vi "Example5-Encapsulation.vi"() -> ()   [LabVIEW 2021]
doc: "Example of object encapsulation in LabVIEW. Comments in Polish."
uses:
  Droid/Droid.lvclass
  Astromech droid/Astromech droid.lvclass
  BB-Series/BB-Series.lvclass
  MedicalDroid/MedicalDroid.lvclass
  BactaTank/BactaTank.lvclass
  BattleDroid/BattleDroid.lvclass
  B1/B1.lvclass
panel:
  out "Output DROID data":cluster{"ID":string, "Active":bool}
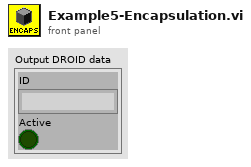
[diagram p1: front panel]
types:
  T1 = cluster{"Mode ":enum16{"GUARD", "RECON", "ATTACK ", "MAINTAINCE"}, "Enviroment Info":variant, "Mission Goals":string[], "DataAboutEnemy":map{string, i32}}
  T2 = enum16{"GUARD", "RECON", "ATTACK ", "MAINTAINCE"}
  T3 = enum16{"Q-Series", "BB-Series", "C-Series", "R-Series"}
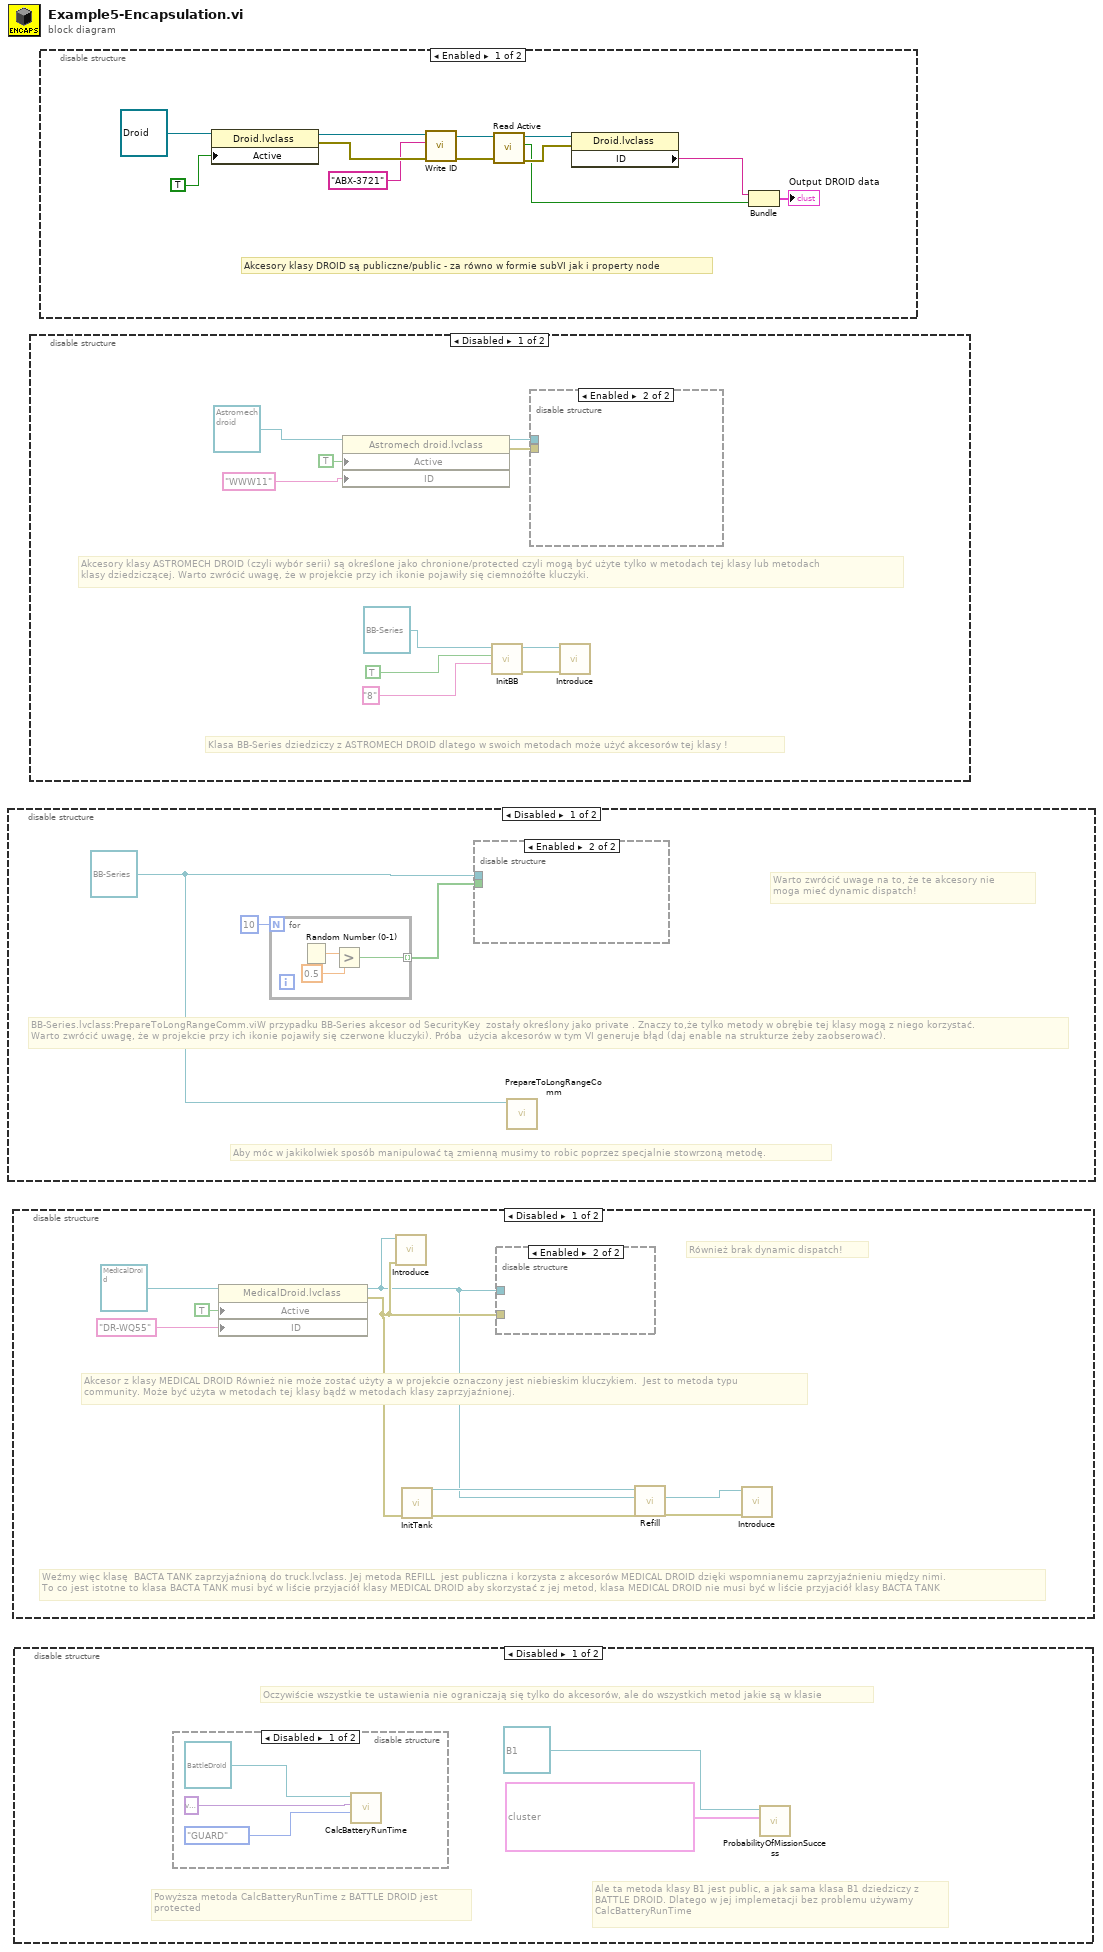
[diagram p0: block diagram]
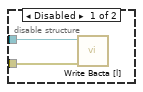
[diagram p4: hidden frame]
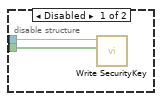
[diagram p6: hidden frame]
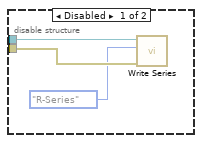
[diagram p8: hidden frame]
diagram:
  n1 = disable-structure shown="Disabled" {
    frame Disabled {
      w1 = refnum<class "BB-Series.lvclass"> refnum ("BB-Series in")
      # "Warto zwrócić uwage na to, że te akcesory nie \nmoga mieć dynamic dispatch!"
      # "Aby móc w jakikolwiek sposób manipulować tą zmienną musimy to robic poprzez specjalnie stowrzoną metodę."
      # "BB-Series.lvclass:PrepareToLongRangeComm.viW przypadku BB-Series akcesor od SecurityKey  zostały określony jako private . Znaczy to,że tylko metody w obrębie tej klasy mogą z niego korzystać. \nWarto zwrócić uwagę, że w projekcie przy ich ikonie pojawiły się czerwone kluczyki). Próba  użycia akcesorów w tym VI generuje błąd (daj enable na strukturze żeby zaobserować)."
      n2 = for {
        N: 10 -> [_]
        tunnel: [w6] -> w2 mode=indexing
        n3 = Random Number (0-1)() -> (number: 0 to 1=w8:dbl)
        n4 = Greater?(x=w8, y=0.5) -> (0:w6:bool)
      }
      n5 = disable-structure shown="Enabled" {
        disable-tunnel: w1 -> [w5 _]
        disable-tunnel: w2 -> [w4 _]
        frame Disabled {
          n6 = call "Write SecurityKey.vi"("SecurityKey"=w4, "BB-Series in"=w5) -> ()  [unwired: 8 in, 2 out]
        }
        frame Enabled {
        }
      }
      n7 = call "PrepareToLongRangeComm.vi"("BB-Series in"=w1) -> ()  [unwired: 9 in, 2 out]
    }
    frame Enabled {
    }
  }
  n8 = disable-structure shown="Disabled" {
    frame Disabled {
      # "Weźmy więc klasę  BACTA TANK zaprzyjaźnioną do truck.lvclass. Jej metoda REFILL  jest publiczna i korzysta z akcesorów MEDICAL DROID dzięki wspomnianemu zaprzyjaźnieniu między nimi. \nTo co jest istotne to klasa BACTA TANK musi być w liście przyjaciół klasy MEDICAL DROID aby skorzystać z jej metod, klasa MEDICAL DROID nie musi być w liście przyjaciół klasy BACTA TANK"
      # "Również brak dynamic dispatch!"
      # "Akcesor z klasy MEDICAL DROID Również nie może zostać użyty a w projekcie oznaczony jest niebieskim kluczykiem.  Jest to metoda typu\ncommunity. Może być użyta w metodach tej klasy bądź w metodach klasy zaprzyjaźnionej."
      n9 = property class="MedicalDroid.lvclass"(reference=refnum<class "MedicalDroid.lvclass"> refnum ("MedicalDroid.lvclass"), "Active"=TRUE, "ID"="DR-WQ55") -> (reference out=w9:refnum<class "MedicalDroid.lvclass">, error out=w10:errorcluster)  [unwired: 1 in]
      n10 = call-dynamic "Introduce.vi"("Error In"=w10, "MedicalDroid in"=w9) -> ()  [unwired: 8 in, 2 out]
      n11 = call "InitTank.vi"("Error In"=w10) -> ("Error Out"=w15:errorcluster, "BactaTank out"=w14:refnum<class "BactaTank.lvclass">)  [unwired: 9 in]
      n12 = disable-structure shown="Enabled" {
        disable-tunnel: w9 -> [w19 _]
        disable-tunnel: w10 -> [w18 _]
        frame Disabled {
          n13 = call "Write Bacta [l].vi"("error in (no error)"=w18, "MedicalDroid in"=w19) -> ()  [unwired: 8 in, 2 out]
        }
        frame Enabled {
        }
      }
      n14 = call "Refill.vi"("Error In"=w15, "MedicalDroid In"=w9, "BactaTank in"=w14) -> ("Error Out"=w17:errorcluster, "MedicalDroid Out"=w16:refnum<class "MedicalDroid.lvclass">)  [unwired: 6 in, 1 out]
      n15 = call-dynamic "Introduce.vi"("Error In"=w17, "MedicalDroid in"=w16) -> ()  [unwired: 8 in, 2 out]
    }
    frame Enabled {
    }
  }
  n16 = disable-structure shown="Disabled" {
    frame Disabled {
      # "Ale ta metoda klasy B1 jest public, a jak sama klasa B1 dziedziczy z\nBATTLE DROID. Dlatego w jej implemetacji bez problemu używamy\nCalcBatteryRunTime"
      # "Powyższa metoda CalcBatteryRunTime z BATTLE DROID jest \nprotected"
      # "Oczywiście wszystkie te ustawienia nie ograniczają się tylko do akcesorów, ale do wszystkich metod jakie są w klasie"
      n17 = disable-structure shown="Disabled" {
        frame Disabled {
          n18 = call "CalcBatteryRunTime.vi"("Mode"=T2."GUARD", "Enviroment Info"=variant, "BattleDroid In"=refnum<class "BattleDroid.lvclass"> refnum) -> ()  [unwired: 6 in, 3 out]
        }
        frame Enabled {
        }
      }
      n19 = call "ProbabilityOfMissionSuccess.vi"("MissionData"=T1 {"Mode "=enum."GUARD", "Enviroment Info"=variant, "Mission Goals"=[], "DataAboutEnemy"={}}, "B1 In"=refnum<class "B1.lvclass"> refnum) -> ()  [unwired: 7 in, 3 out]
    }
    frame Enabled {
    }
  }
  n20 = disable-structure shown="Disabled" {
    frame Disabled {
      # "Klasa BB-Series dziedziczy z ASTROMECH DROID dlatego w swoich metodach może użyć akcesorów tej klasy !"
      # "Akcesory klasy ASTROMECH DROID (czyli wybór serii) są określone jako chronione/protected czyli mogą być użyte tylko w metodach tej klasy lub metodach\nklasy dziedziczącej. Warto zwrócić uwagę, że w projekcie przy ich ikonie pojawiły się ciemnożółte kluczyki."
      n21 = property class="Astromech droid.lvclass"(reference=refnum<class "Astromech droid.lvclass"> refnum ("Astromech droid.lvclass"), "Active"=TRUE, "ID"="WWW11") -> (reference out=w31:refnum<class "Astromech droid.lvclass">, error out=w30:errorcluster)  [unwired: 1 in]
      n22 = call "InitBB.vi"("ID"="8", "Active"=TRUE, "BB-Series in"=refnum<class "BB-Series.lvclass"> refnum) -> ("Error Out"=w27:errorcluster, "BB-Series out"=w28:refnum<class "BB-Series.lvclass">)  [unwired: 7 in]
      n23 = disable-structure shown="Enabled" {
        disable-tunnel: w31 -> [w37 _]
        disable-tunnel: w30 -> [w36 _]
        frame Disabled {
          n24 = call-dynamic "Write Series.vi"("error in (no error)"=w36, "Series"=T3."R-Series", "Astromech droid in"=w37) -> ()  [unwired: 7 in, 2 out]
        }
        frame Enabled {
        }
      }
      n25 = call-dynamic "Introduce.vi"("Error In"=w27, "BB-Series in"=w28) -> ()  [unwired: 8 in, 2 out]
    }
    frame Enabled {
    }
  }
  n26 = disable-structure shown="Enabled" {
    frame Enabled {
      # "Akcesory klasy DROID są publiczne/public - za równo w formie subVI jak i property node"
      n27 = property class="Droid.lvclass"(reference=refnum<class "Droid.lvclass"> refnum ("Droid.lvclass"), "Active"=TRUE) -> (reference out=w47:refnum<class "Droid.lvclass">, error out=w46:errorcluster)  [unwired: 1 in]
      n28 = call-dynamic "Write ID.vi"("error in (no error)"=w46, "ID"="ABX-3721", "Droid in"=w47) -> ("error out"=w43:errorcluster, "Droid out"=w44:refnum<class "Droid.lvclass">)  [unwired: 7 in]
      n29 = call-dynamic "Read Active.vi"("error in (no error)"=w43, "Droid in"=w44) -> ("error out"=w41:errorcluster, "Active"=w39:bool, "Droid out"=w42:refnum<class "Droid.lvclass">)  [unwired: 7 in]
      n30 = property class="Droid.lvclass"(reference=w42, error in=w41) -> ("ID"=w40:string)  [unwired: 2 out]
      n31 = Bundle("ID"=w40, "Active"=w39) -> (→"Output DROID data":cluster{"ID":string, "Active":bool})  [unwired: 1 in]
    }
    frame Disabled {
    }
  }
